vi "Report Generation Print Barcode.vi"() -> ()   [LabVIEW 2013]
uses:
  <vilib>/Utility/NIReport.llb/NI_report.lvclass
  <vilib>/Utility/NIReport.llb/Append Report Text (str wrap).vi
panel:
  in  "error in (no error)":errorcluster
  out "error out":errorcluster
  in  "printer name (default)":string
  in  "font settings":T1={"Charset (-1)"=-1, "Weight (-1)"=-1, "Name"="", "Size"=" "}
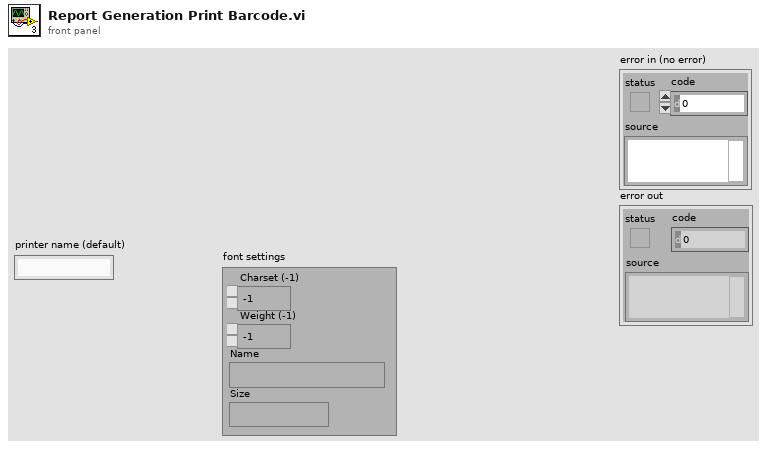
[diagram p1: front panel]
types:
  T1 = cluster{"Charset (-1)":i16, "Weight (-1)":i16, "Name":string, "Size":string}
  T2 = enum16{"Standard Report", "HTML", "Word", "Excel"}
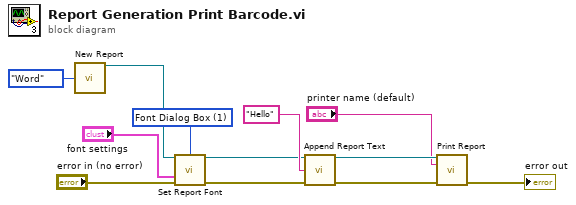
[diagram p0: block diagram]
diagram:
  w9 = u16 1 items=["VI Inputs", "Font Dialog Box"] ("font settings source")
  n1 = call <vilib>:"New Report.vi"("report type"=T2."Word") -> ("report out"=w6:refnum<class "NI_report.lvclass">)  [unwired: 13 in, 1 out]
  n2 = call-dynamic "Set Report Font.vi"("report in"=w6, "font settings source (VI Inputs)"=w9, "font settings"="font settings", "error in (no error)"="error in (no error)") -> ("report out"=w5:refnum<class "NI_report.lvclass">, "error out"=w4:errorcluster)  [unwired: 9 in, 1 out]
  n3 = call-poly <vilib>:"Append Report Text.vi"("report in"=w5, "text"="Hello", "error in (no error)"=w4) -> ("report out"=w3:refnum<class "NI_report.lvclass">, "error out"=w2:errorcluster)  [unwired: 9 in, 2 out]
  n4 = call-dynamic "Print Report.vi"("report in"=w3, "printer name (default)"="printer name (default)", "error in (no error)"=w2) -> ("error out"=→"error out":errorcluster)  [unwired: 11 in, 1 out]
